vi "LASER_Clear.vi"(8 "error in":errorcluster, 11 "Constant Output Configuration":T1) -> (0 "error out":errorcluster)   [LabVIEW 2010]
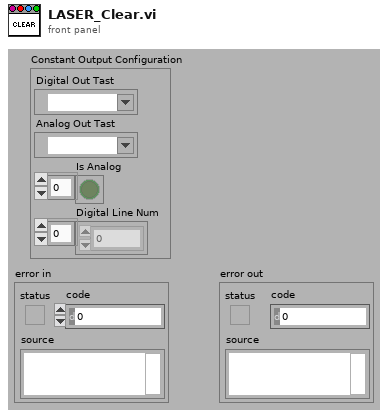
[diagram p1: front panel]
types:
  T1 = cluster{"Digital Out Tast":refnum<k21>, "Analog Out Tast":refnum<k21>, "Is Analog":bool[], "Digital Line Num":u32[]}
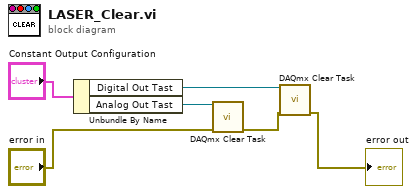
[diagram p0: block diagram]
diagram:
  n1 = Unbundle By Name("Constant Output Configuration") -> ("Digital Out Tast"=w5:refnum<k21>, "Analog Out Tast"=w4:refnum<k21>)
  n2 = call <vilib>:"DAQmx Clear Task.vi"("task in"=w4, "error in"="error in") -> ("error out"=w2:errorcluster)  [unwired: 13 in]
  n3 = call <vilib>:"DAQmx Clear Task.vi"("task in"=w5, "error in"=w2) -> ("error out"=→"error out":errorcluster)  [unwired: 13 in]
